vi "Sweep Control.vi"(0 "Scan control":T12=[{"Priority"=enum."Priority 1", "Scan name"=enum."OFF"}, {"Priority"=enum."Priority 0", "Scan name"=enum."DSA_freq"}, {"Priority"=enum."Priority 3", "Scan name"=enum."OFF"}, {"Priority"=enum."Priority 2", "Scan name"=enum."OFF"}], 1 "Scan parameters":T10=[{"DAQ Channel"=0, "Label"="\nappliedDC=", "Start"=-0.00372, "End"=0.00428, "Step"=5e-05, "Rate"=0.0, "VISA resource name"="", "wait (ms)"=10000}, {"DAQ Channel"=3, "Label"="\nappliedField=", "Start"=0.3, "End"=0.0, "Step"=0.02, "Rate"=0.05, "VISA resource name"="", "wait (ms)"=10000}, {"DAQ Channel"=3, "Label"="\nappliedVbg=", "Start"=-1.55, "End"=3.0, "Step"=0.015, "Rate"=2.0, "VISA resource name"="", "wait (ms)"=10000}, {"DAQ Channel"=3, "Label"="\nappliedField=", "Start"=0.0, "End"=10000.0, "Step"=5000.0, "Rate"=0.0, "VISA resource name"="", "wait (ms)"=10000}] {"Rate" format="%.2f"; "Step" format="%#_6p"; "End" format="%#_6p"; "Start" format="%#_6p"}, 4 "Experiment folder name":string="21-SmallBsweep-DCsweep-rightdrive12-leftgrounded") -> ()   [LabVIEW 2016, in "SweepControl.lvclass"]
uses:
  SweepControl.lvclass
  Typedefs/ScanControl.ctl
  Typedefs/Cluster - ScanControl.ctl
  Typedefs/Enum - Priority.ctl
  Typedefs/Enum - Action.ctl
  Typedefs/ScanParamters.ctl
  Typedefs/Cluster - ScanParamters.ctl
  Typedefs/PostAction.ctl
  Typedefs/Enum - PostAction.ctl
  <userlib>/LevyLab/Lockin-Multichannel/Typedefs/AO-cluster.ctl
  <userlib>/LevyLab/Lockin-Multichannel/Typedefs/AO_Amp-array.ctl
  <userlib>/LevyLab/Lockin-Multichannel/Typedefs/AO_DC-array.ctl
  <userlib>/LevyLab/Lockin-Multichannel/Typedefs/AO_f-array.ctl
  <userlib>/LevyLab/Lockin-Multichannel/Typedefs/AO_phi-array.ctl
  <userlib>/LevyLab/Lockin-Multichannel/Typedefs/Function-array.ctl
  <userlib>/LevyLab/Lockin-Multichannel/Typedefs/Function-enum.ctl
  SweepControl.lvclass/SweepControl.ctl
  Transport.lvclass
panel:
  in  "Comments":string
  in  "Channels: AO":T1={"AO amp (V)"=[0.0002, 0.0, 0.0, 0.0, 0.0, 0.0, 0.0, 0.0], "AO DC (V)"=[-0.004, 0.0, 0.04, 0.0, 0.0, 0.0, 0.0, 0.0], "AO f (Hz)"=[9.0, 3.0, 3.0, 3.0, 3.0, 3.0, 3.0, 3.0], "AO phi (deg)"=[0.0, 0.0, 0.0, 0.0, 0.0, 0.0, 0.0, 0.0], "function"=[enum."Sine Wave", enum."Sine Wave", enum."Sine Wave", enum."Sine Wave", enum."Sine Wave", enum."Sine Wave", enum."Sine Wave", enum."Sine Wave"]} {"AO f (Hz)" min=0.001 max=10000.0; "AO DC (V)" format="%#_6p"; "AO amp (V)" format="%#_6p"}
  in  "Experiment":enum16{"IV", "lockin_time", "Lockin_Vsg"}(ring)=enum."Lockin_Vsg"
  in  "Post action (indexing priority)":T8=[enum."Do Nothing", enum."Wait", enum."Do Nothing", enum."Do Nothing"]
  in  "Experiments @ each parameter":i32=1
  # "if you use the lockin\nprogram remember to\nset BG/SG parameters in\n'lockin_Vsg_multichannel.vi'"
  # "Instructions: \n1, you can put multiple scan names in one priority.\n2 OFF has to put in last priority"
  # "0"
  # "1"
  # "2"
  # "3"
  # "4"
  # "5"
  # "6"
  # "7"
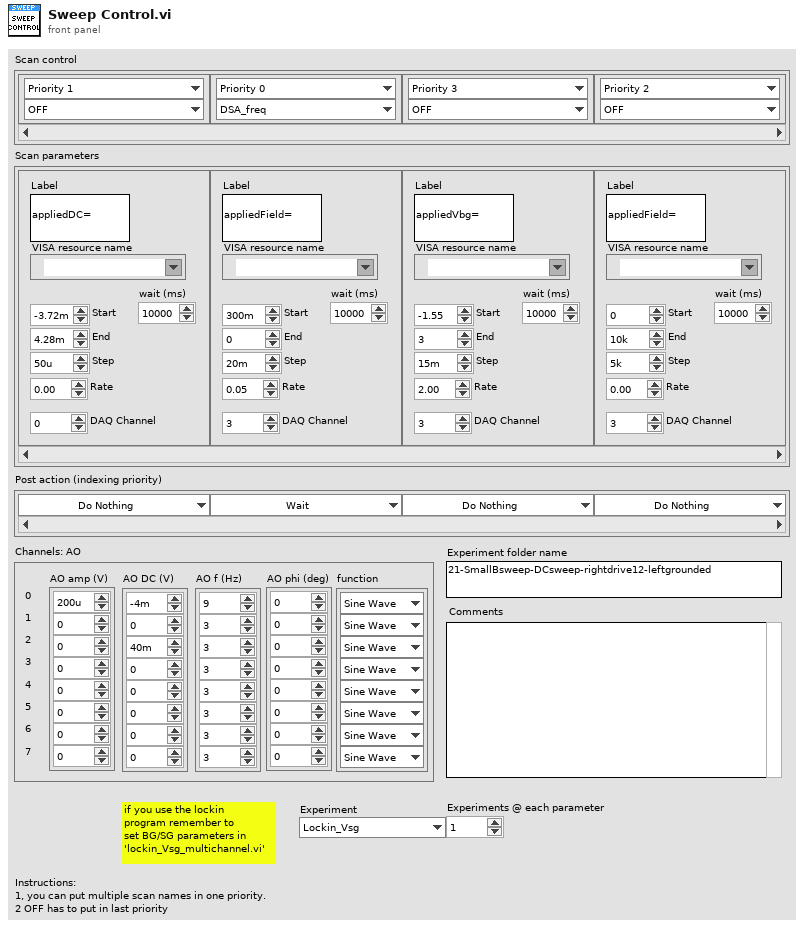
[diagram p1: front panel]
types:
  T1 = typedef "AO-cluster.ctl" = cluster{"AO amp (V)":T2, "AO DC (V)":T3, "AO f (Hz)":T4, "AO phi (deg)":T5, "function":T6}
  T2 = typedef "AO_Amp-array.ctl" = dbl[]
  T3 = typedef "AO_DC-array.ctl" = dbl[]
  T4 = typedef "AO_f-array.ctl" = dbl[]
  T5 = typedef "AO_phi-array.ctl" = dbl[]
  T6 = typedef "Function-array.ctl" = T7[]
  T7 = typedef "Function-enum.ctl" = enum16{"Sine Wave", "Triangle Wave", "Square Wave", "Sawtooth Wave"}
  T8 = typedef "SweepControl.lvclass/PostAction.ctl" = T9[]
  T9 = typedef "SweepControl.lvclass/Enum - PostAction.ctl" = enum16{"Clear DAQ Tasks", "Check Temperature", "Wait", "Do Nothing"}
  T10 = typedef "SweepControl.lvclass/ScanParamters.ctl" = T11[]
  T11 = typedef "SweepControl.lvclass/Cluster - ScanParamters.ctl" = cluster{"DAQ Channel":i32, "Label":string, "Start":dbl, "End":dbl, "Step":dbl, "Rate":dbl, "VISA resource name":refnum<visa-resource-name>, "wait (ms)":u32}
  T12 = typedef "SweepControl.lvclass/ScanControl.ctl" = T13[]
  T13 = typedef "SweepControl.lvclass/Cluster - ScanControl.ctl" = cluster{"Priority":T14, "Scan name":T15}
  T14 = typedef "SweepControl.lvclass/Enum - Priority.ctl" = enum16{"Priority 0", "Priority 1", "Priority 2", "Priority 3", "Priority 4", "Priority 5"}
  T15 = typedef "SweepControl.lvclass/Enum - Action.ctl" = enum16{"OFF", "DSA_Vamp", "DSA_freq", "DSA_Vsg1", "DSA_Vsg2", "DSA_Vsg3", "DAQ_Vbg", "B_Field", "Humidity", "Temp", "MW_freq1", "MW_freq2", "MW_amplitude1", "MW_amplitude2"}
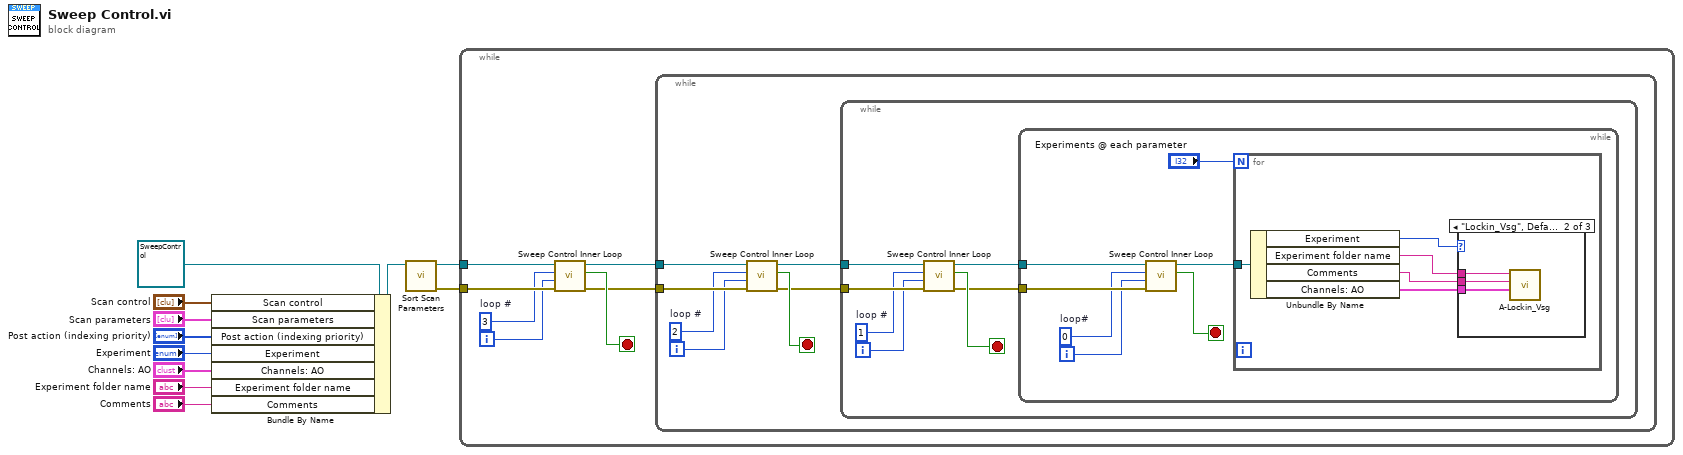
[diagram p0: block diagram]
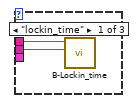
[diagram p2: hidden frame]
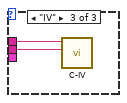
[diagram p3: hidden frame]
diagram:
  n1 = Bundle By Name(cluster=refnum<class "SweepControl.lvclass"> refnum ("SweepControl.lvclass"), "Scan control"="Scan control", "Scan parameters"="Scan parameters", "Post action (indexing priority)"="Post action (indexing priority)", "Experiment"="Experiment", "Channels: AO"="Channels: AO", "Experiment folder name"="Experiment folder name", "Comments"="Comments") -> (w10:refnum<class "SweepControl.lvclass">)
  n2 = call "Sort Scan Parameters.vi"("SweepControl"=w10) -> ("error out"=w7:errorcluster, "SweepControl"=w8:refnum<class "SweepControl.lvclass">)  [unwired: 7 in, 2 out]
  n3 = while {
    tunnel: w8 -> [w17]
    tunnel: w7 -> [w15]
    i -> [w14]
    stop <- w18 stop-if-true
    w13 = 3  # loop #
    n4 = call "Sweep Control Inner Loop.vi"("error in (no error)"=w15, "index"=w14, "loop #"=w13, "SweepControl in"=w17) -> ("error out"=w12:errorcluster, "Stop?"=w18:bool, "SweepControl out"=w16:refnum<class "SweepControl.lvclass">)  [unwired: 5 in]
    n5 = while {
      tunnel: w16 -> [w25]
      tunnel: w12 -> [w24]
      i -> [w22]
      stop <- w21 stop-if-true
      w23 = 2  # loop #
      n6 = call "Sweep Control Inner Loop.vi"("error in (no error)"=w24, "index"=w22, "loop #"=w23, "SweepControl in"=w25) -> ("error out"=w20:errorcluster, "Stop?"=w21:bool, "SweepControl out"=w19:refnum<class "SweepControl.lvclass">)  [unwired: 5 in]
      n7 = while {
        tunnel: w20 -> [w32]
        tunnel: w19 -> [w31]
        i -> [w29]
        stop <- w28 stop-if-true
        w30 = 1  # loop #
        n8 = call "Sweep Control Inner Loop.vi"("error in (no error)"=w32, "index"=w29, "loop #"=w30, "SweepControl in"=w31) -> ("error out"=w27:errorcluster, "Stop?"=w28:bool, "SweepControl out"=w26:refnum<class "SweepControl.lvclass">)  [unwired: 5 in]
        n9 = while {
          tunnel: w27 -> [w38]
          tunnel: w26 -> [w37]
          i -> [w35]
          stop <- w34 stop-if-true
          w36 = 0  # loop#
          n10 = call "Sweep Control Inner Loop.vi"("error in (no error)"=w38, "index"=w35, "loop #"=w36, "SweepControl in"=w37) -> ("Stop?"=w34:bool, "SweepControl out"=w33:refnum<class "SweepControl.lvclass">)  [unwired: 5 in, 1 out]
          n11 = for {
            N: "Experiments @ each parameter" -> [_]
            tunnel: w33 -> [w40]
            n12 = Unbundle By Name(w40) -> ("Experiment"=w43:enum16{"IV", "lockin_time", "Lockin_Vsg"}, "Experiment folder name"=w42:string, "Comments"=w41:string, "Channels: AO"=w44:T1)
            n13 = case shown="\"Lockin_Vsg\", Default" w43 {
              tunnel: w42 -> [w46 w49 w51]
              tunnel: w41 -> [w45 w48 w50]
              tunnel: w44 -> [_ w47 _]
              frame "lockin_time" {
                n14 = call "B-Lockin_time.vi"("Comments"=w45, "folder name"=w46) -> ()  [unwired: 7 in, 3 out]
              }
              frame "Lockin_Vsg", Default {
                n15 = call "A-Lockin_Vsg.vi"("Channels: AO"=w47, "Comments"=w48, "ITX folder"=w49) -> ()  [unwired: 9 in]
              }
              frame "IV" {
                n16 = call "C-IV.vi"("Notes 2"=w50, "Experiment folder name"=w51) -> ()  [unwired: 8 in, 2 out]
              }
            }
          }
        }
      }
    }
  }
